vi "XIPIN_IOModule_3_0.vi"   [LabVIEW 2017]
doc: "LMB module which includes plenty of I/O peripherals\n------------------------------------\n<b>Need License</b> : No"
uses:
  <vilib>/rvi/XilinxIP/XIPIN_XNode/niFpgaXIPIN.xnode
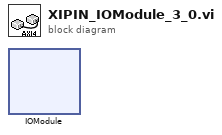
[diagram p0: block diagram]
diagram:
  n1 = xnode ("IOModule")() -> ()
